vi "Set Server Address.vi"(10 "Server Address":string, 11 "OOP Server in":refnum<class "MeasurementService_Template.lvclass">) -> (3 "OOP Server out":refnum<class "MeasurementService_Template.lvclass">)   [LabVIEW 2020, in "MeasurementService_Template.lvlib" / "MeasurementService_Template.lvclass"]
uses:
  MeasurementService_Template.lvclass
  MeasurementService_Template.lvclass/MeasurementService_Template.ctl
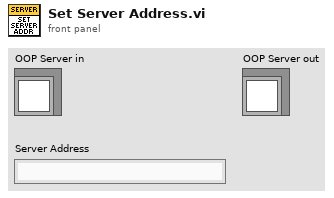
[diagram p1: front panel]
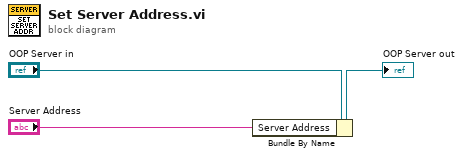
[diagram p0: block diagram]
diagram:
  n1 = Bundle By Name(cluster="OOP Server in", "Server Address"="Server Address") -> (→"OOP Server out":refnum<class "MeasurementService_Template.lvclass">)
